vi "Open URL in Default Browser (path).vi"(4 "error in (no error)":errorcluster, 7 "path":path) -> (0 "error out":errorcluster, 3 "URL out":string)   [LabVIEW 2015]
doc: "Displays a URL or HTML file in the default Web browser. If the URL or path you wire to this VI contains a space character, the VI encodes the space as %20 before displaying the URL or HTML file in the Web browser. Wire data to the <B>URL</B> input to determine the polymorphic instance to use or manually select the instance."
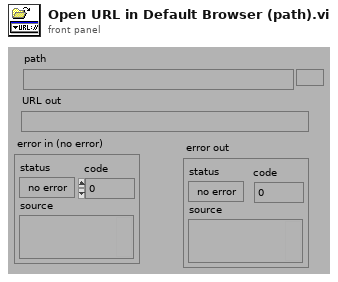
[diagram p1: front panel]
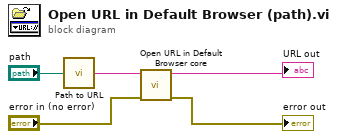
[diagram p0: block diagram]
diagram:
  n1 = call "Path to URL.vi"("path"="path") -> ("url"=w4:string)
  n2 = call "Open URL in Default Browser core.vi"("error in (no error)"="error in (no error)", "url"=w4) -> ("error out"=→"error out":errorcluster, "duplicate url"=→"URL out":string)  [unwired: 4 in]
